vi "c_ctre_phoenix6_RequestControlCoastOut.vi"(0 "String":string, 1 "Numeric 2":u32, 2 "Numeric 3":dbl, 3 "Numeric 4":u8) -> (20 "Numeric":i32)   [LabVIEW 2023]
uses:
  <vilib>/Rock Robotics/WPI/ThirdParty/Phoenix-LabVIEW/Controls/DriverLib.ctl
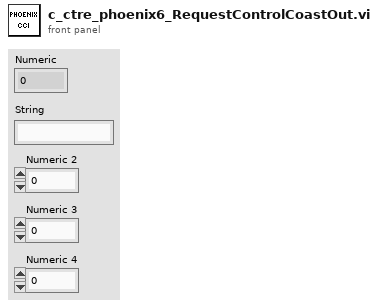
[diagram p1: front panel]
types:
  T1 = typedef "DriverLib.ctl" = path
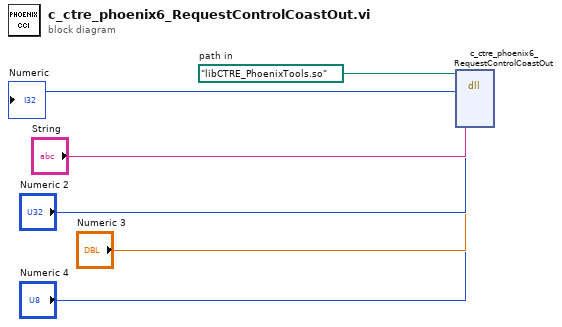
[diagram p0: block diagram]
diagram:
  w6 = T1 path "libCTRE_PhoenixTools.so"  # path in
  n1 = dll-call lib="?" fn="c_ctre_phoenix6_RequestControlCoastOut"(path in=w6, "String", "Numeric 2", "Numeric 3", "Numeric 4") -> (→"Numeric":i32)  [unwired: 6 in, 2 out]
